vi "stop_hp_test_if_gb_test_fail.vi"(8 "error in (no error)":errorcluster, 9 "Message Queues in":T1, 11 "Pass/Fail":cluster{"PASS":bool, "FAIL":bool}) -> (0 "error out":errorcluster, 2 "Stop":bool)   [LabVIEW 2015]
uses:
  support/Message Queue/All Message Queues.ctl
  support/Message Queue/Message Cluster.ctl
  support/Message Queue/Enqueue Message (Array).vi
  support/Message Queue/Message Queue.lvlib
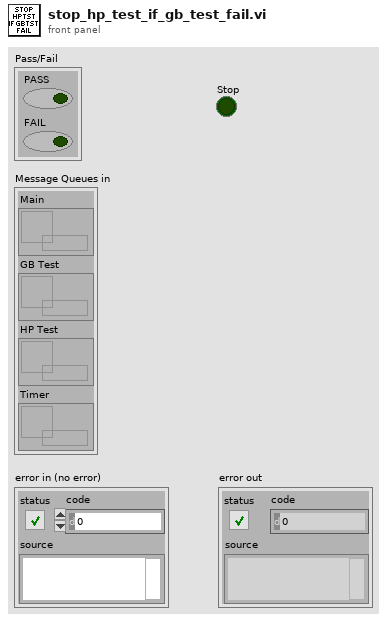
[diagram p1: front panel]
types:
  T1 = typedef "Message Queue.lvlib/All Message Queues.ctl" = cluster{"Main":refnum<queue>, "GB Test":refnum<queue>, "HP Test":refnum<queue>, "Timer":refnum<queue>}
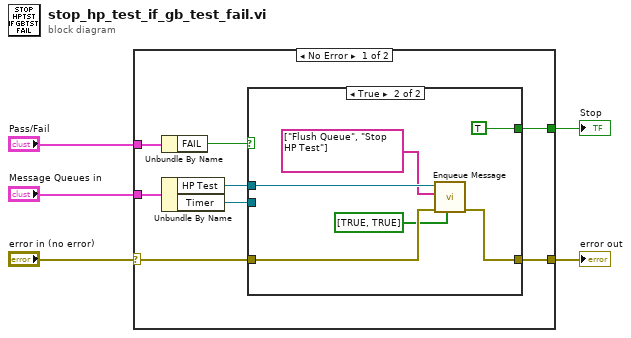
[diagram p0: block diagram]
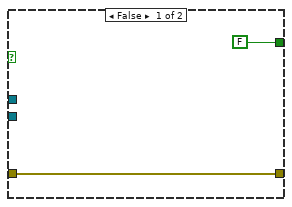
[diagram p2: hidden frame]
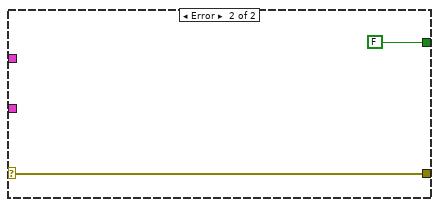
[diagram p3: hidden frame]
diagram:
  n1 = case shown="No Error" "error in (no error)" {
    selector: "error in (no error)" -> [w8 w23]
    tunnel: "Pass/Fail" -> [w12 _]
    tunnel: "Message Queues in" -> [w11 _]
    tunnel: [w7 w23] -> w2
    tunnel: [w6 FALSE] -> w1
    frame No Error {
      n2 = Unbundle By Name(w12) -> ("FAIL"=w13:bool)
      n3 = Unbundle By Name(w11) -> ("HP Test"=w10:refnum<queue>, "Timer"=w9:refnum<queue>)
      n4 = case shown="True" w13 {
        tunnel: w10 -> [_ w21]
        tunnel: w9 -> [_ _]
        tunnel: w8 -> [w15 w19]
        tunnel: [w15 w16] -> w7
        tunnel: [FALSE TRUE] -> w6
        frame False {
        }
        frame True {
          n5 = call-poly "Enqueue Message.vi"("Priority Message? Array"=bool[] [TRUE, TRUE], "error in (no error)"=w19, "Message Array"=string[] ["Flush Queue", "Stop HP Test"], "Message Queue"=w21) -> ("error out"=w16:errorcluster)  [unwired: 6 in, 1 out]
        }
      }
    }
    frame Error {
    }
  }
  "error out" <- w2
  "Stop" <- w1
